vi "Read Limit.vi"(8 "error in (no error)":errorcluster, 11 "Analog-Output in":refnum<class "Analog-Output.lvclass">) -> (0 "error out":errorcluster, 2 "Limit":cluster{"Max_V":dbl, "Min_V":dbl}, 3 "Analog-Output out":refnum<class "Analog-Output.lvclass">)   [LabVIEW 2019, in "Analog-Output.lvlib" / "Analog-Output.lvclass"]
uses:
  Library/Analog-Output.lvclass
  Library/Analog-Output.lvclass/Analog-Output.ctl
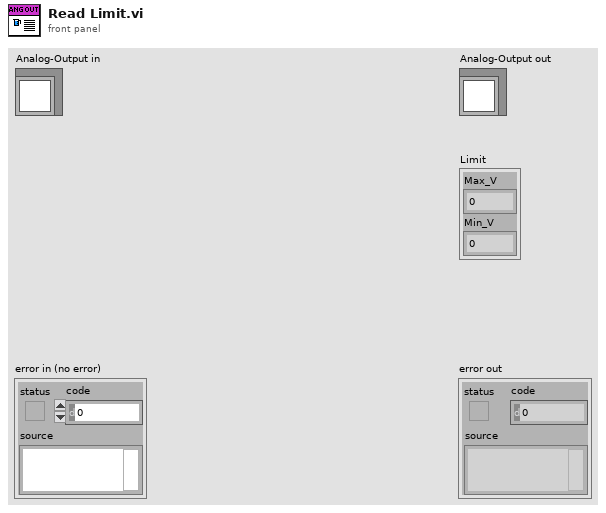
[diagram p1: front panel]
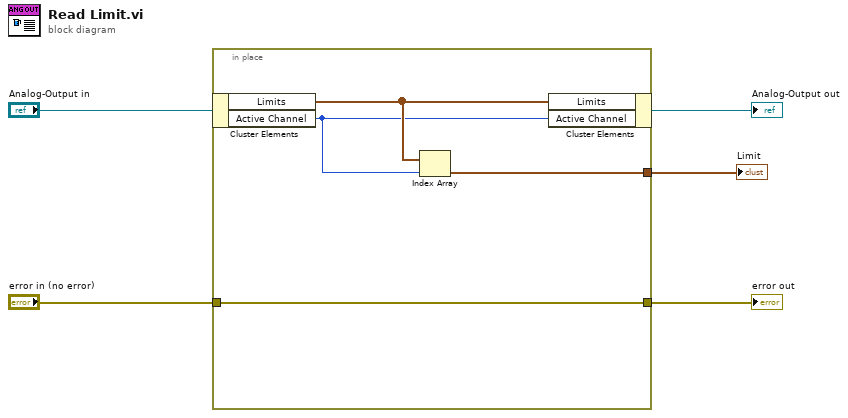
[diagram p0: block diagram]
diagram:
  n1 = in-place {
    in-place-border: [w7] -> w4
    in-place-border: [w6] -> w3
    in-place-border: "error in (no error)" -> [w6]
    n2 = in-place-cluster #1("Analog-Output in") -> ("Limits"=w9:cluster{"Max_V":dbl, "Min_V":dbl}[], "Active Channel"=w8:u32)
    n3 = Index Array(array=w9, index=w8) -> (element=w7:cluster{"Max_V":dbl, "Min_V":dbl})
    n4 = in-place-cluster #1("Limits"=w9, "Active Channel"=w8) -> (→"Analog-Output out":refnum<class "Analog-Output.lvclass">)
  }
  "error out" <- w3
  "Limit" <- w4
